vi "F2ToFalseColor.vi"(1 "Intensity":u32[][][][](array[numeric]), 2 "Plane":u32, 3 "Threshold (max)":cluster{"max":u32, "min":u32}) -> (0 "FalseColor":u32[][](array[numeric]))   [LabVIEW 2009]
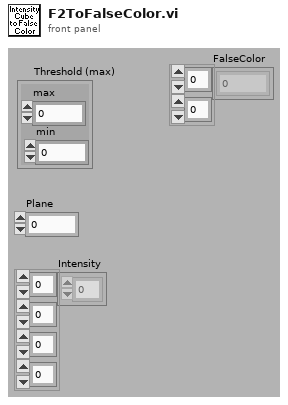
[diagram p1: front panel]
types:
  T1 = typedef "Settings.ctl" = cluster{"threshold":cluster{"max":u32, "min":u32}, "RGB or false color":bool, "16bit":bool, "log/lin axis":u16, "spotsize button":bool, "Pixelsize":u16, "autoscale x":bool, "autoscale y":bool, "correlation":bool, "ADC-Resolution":i32, "F2-lifetime":cluster{"display tau":bool, "display F2":bool, "Palette Number lifetime":enum32{"Gray", "Binary", "Gradient", "Rainbow", "Temperature"}, "Palette Number F2":enum32{"Gray", "Binary", "Gradient", "Rainbow", "Temperature"}, "max tau-Value":dbl, "min tau-Value":dbl, "max F2-Value":dbl, "min F2-Value":dbl}, "TAC-Window 1":u16, "TAC-Window 2":u16, "false color palette":cluster{"1":u32, "2":u32, "3":u32, "4":u32, "5":u32, "6":u32, "7":u32, "8":u32, "8 2":u32, "8 3":u32, "8 4":u32, "8 5":u32}}
  T2 = cluster{"1":u32, "2":u32, "3":u32, "4":u32, "5":u32, "6":u32, "7":u32, "8":u32, "8 2":u32, "8 3":u32, "8 4":u32, "8 5":u32}
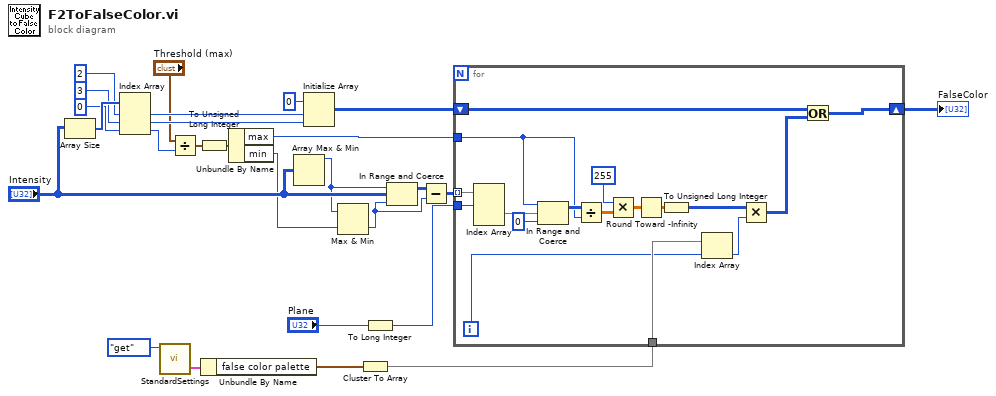
[diagram p0: block diagram]
diagram:
  n1 = Array Size(array="Intensity") -> (size(s)=w23:i32[])
  n2 = Index Array(array=w23, index #1=2 ("index"), index #2=3 ("index"), index #3=0 ("index")) -> (element #1=w18:i32, element #2=w17:i32, element #3=w13:i32)
  n3 = call "StandardSettings.vi"("Enum"=enum16{"Load", "get", "Save", "set"}."get") -> ("StandardSettings"=w7:T1)  [unwired: 4 in]
  n4 = Divide(x="Threshold (max)", y=w13) -> (x/y=w11:cluster{"max":dbl, "min":dbl})
  n5 = To Unsigned Long Integer(number=w11) -> (unsigned 32bit integer=w10:cluster{"max":u32, "min":u32})
  n6 = Unbundle By Name(w7) -> ("false color palette"=w6:T2)
  n7 = Unbundle By Name(w10) -> ("max"=w9:u32, "min"=w3:u32)
  n8 = Array Max & Min(array="Intensity") -> (max value=w2:u32)  [unwired: 3 out]
  n9 = Initialize Array(u32 0, w18, w17) -> (w20:u32[][])
  n10 = Max & Min(x=w2, y=w3) -> (min(x,y)=w1:u32)  [unwired: 1 out]
  n11 = Cluster To Array(cluster=w6) -> (array=w5:u32[])
  n12 = To Long Integer(number="Plane") -> (32bit integer=w4:i32)
  n13 = In Range and Coerce(upper limit=w2, x="Intensity", lower limit=w1) -> (coerced(x)=w16:u32[][][][])  [unwired: 1 out]
  n14 = Subtract(x=w16, y=w1) -> (x-y=w15:u32[][][][])
  n15 = for {
    tunnel: w15 -> [w43] mode=indexing
    tunnel: w4 -> [w42]
    shift-right: [w33] -> w26
    shift-left: w20 -> [w28]
    tunnel: w9 -> [w34]
    tunnel: w5 -> [w30]
    i -> [w29]
    n16 = Index Array(array=w43, index (dim 0)=w42) -> (element=w41:u32[][])  [unwired: 2 in]
    n17 = In Range and Coerce(upper limit=w34, x=w41, lower limit=u32 0) -> (coerced(x)=w39:u32[][])  [unwired: 1 out]
    n18 = Divide(x=w39, y=w34) -> (x/y=w38:dbl[][])
    n19 = Multiply(x=u32 255 ("Threshold (max)"), y=w38) -> (x*y=w36:dbl[][])
    n20 = Round Toward -Infinity(1:w36) -> (0:w35:dbl[][])
    n21 = To Unsigned Long Integer(number=w35) -> (unsigned 32bit integer=w32:u32[][])
    n22 = Index Array(array=w30, index=w29) -> (element=w31:u32)
    n23 = Multiply(x=w32, y=w31) -> (x*y=w27:u32[][])
    n24 = Or(x=w28, y=w27) -> (x .or. y?=w33:u32[][])
  }
  "FalseColor" <- w26
